vi "SMU_ Set Source Delay.vi"(5 "Source Delay":dbl=0.001, 8 "error in (no error)":errorcluster, 10 "Pins":string[](array[string]), 11 "Semiconductor Module Context":T1) -> (0 "error out":errorcluster, 3 "Source Delay Readback":dbl)   [LabVIEW 2013]
uses:
  <vilib>/NI_TestStand_SemiconductorModule/NI_TestStand_Semiconductor_Module.lvlibp/PinMap/General/SemiconductorModuleContext.ctl
  <vilib>/NI_TestStand_SemiconductorModule/NI_TestStand_Semiconductor_Module.lvlibp/PinMap/DC Power/PinsToNIDCPowerSessions.vi
  <vilib>/NI_TestStand_SemiconductorModule/NI_TestStand_Semiconductor_Module.lvlibp
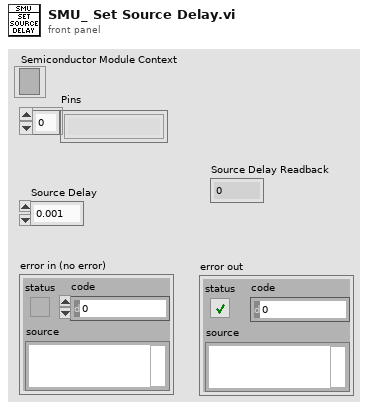
[diagram p1: front panel]
types:
  T1 = typedef "NI_TestStand_Semiconductor_Module.lvlibp/SemiconductorModuleContext.ctl" = refnum<k7>
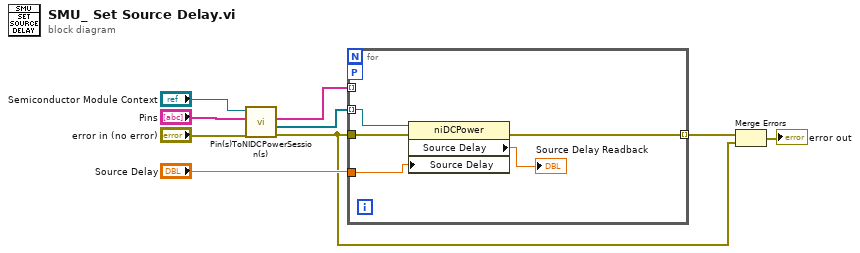
[diagram p0: block diagram]
diagram:
  n1 = call-poly <vilib>:"Pin(s)ToNIDCPowerSession(s).vi"("error in (no error)"="error in (no error)", "Pins"="Pins", "Semiconductor Module Context"="Semiconductor Module Context") -> ("error out"=w2:errorcluster, "Instrument Sessions"=w7:refnum<k15>[], "Channel Lists"=w6:string[])  [unwired: 4 in, 2 out]
  n2 = for {
    tunnel: w7 -> [w14] mode=indexing
    tunnel: w6 -> [_] mode=indexing
    tunnel: "Source Delay" -> [w11]
    tunnel: w2 -> [w13]
    tunnel: [w12] -> w4 mode=indexing
    workers-P: _ -> [_]
    n3 = property class="niDCPower"(reference=w14, error in=w13, "Source Delay"=w11) -> (error out=w12:errorcluster, "Source Delay"=→"Source Delay Readback":dbl)  [unwired: 1 out]
  }
  n4 = Merge Errors(w4, w2) -> (→"error out":errorcluster)
